vi "Network-String to Length-Prefixed Byte Array.vi"(7 "String":string, 13 "byte order":T1(ring)=enum."little-endian") -> (8 "String":string)   [LabVIEW 2020]
panel:
  out "unsigned byte array":u8[](array[numeric])
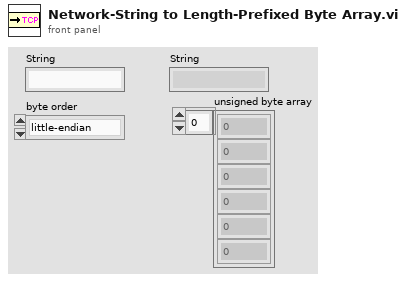
[diagram p1: front panel]
types:
  T1 = enum16{"big-endian, network order", "native, host order", "little-endian"}
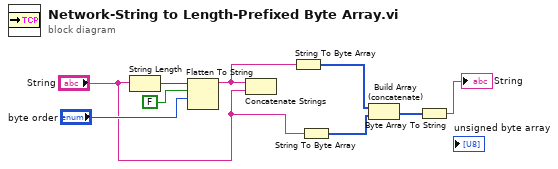
[diagram p0: block diagram]
diagram:
  n1 = String Length(string="String") -> (length=w7:i32)
  n2 = Flatten To String(anything=w7, prepend array or string size? (T)=FALSE, byte order (0:big-endian, network order)="byte order") -> (data string=w5:string)  [unwired: 1 in, 2 out]
  n3 = Concatenate Strings(w5, "String") -> ()  [unwired: 1 out]
  n4 = String To Byte Array(string=w5) -> (unsigned byte array=w4:u8[])
  n5 = String To Byte Array(string="String") -> (unsigned byte array=w3:u8[])
  n6 = Build Array (concatenate)(w4, w3) -> (w2:u8[])
  n7 = Byte Array To String(unsigned byte array=w2) -> (string=→"String":string)
